vi "processamento_deteccao_frequencia_natural_vibracao.vi"() -> ()   [LabVIEW 2011]
uses:
  <vilib>/measure/NI_MAPro.lvlib
  <vilib>/measure/mamon.llb/Waveform Peak Detection for 1 Chan.vi
  <vilib>/measure/maspectr.llb/FFT Spectrum (Mag-Phase) for 1 Chan.vi
panel:
  out "x/y":dbl[](array[numeric])
  in  "Coluna":i32
  out "x-y":dbl
  out "direito 2":dbl
  out "esquerdo 2":dbl
  in  "Frequência de amostragem":dbl
  out "?":waveform(dbl)(graph)
  out "direito":dbl
  out "esquerdo":dbl
  out "Espectro de frequência (detalhado)":cluster{"Y":dbl[], "Y":dbl[]}[](graph)
  out "Picos de frequência\n(frequência, amplitude)":dbl[][](array[numeric])
  out "Espectro de frequência":cluster{"f0":dbl, "df":dbl, "magnitude":dbl[]}(graph)
  in  "stop":bool
  in  "Abrir arquivo":path
  # "PROGRAMA DE IDENTIFICAÇÃO DE \nFREQUÊNCIA NATURAL DE VIBRAÇÃO"
  # "Desenvolvido por\nEloi Antonio Triaca"
  # "*É recomendável que o cursor esquerdo (amarelo) permaneça na posição \"X =0\" ."
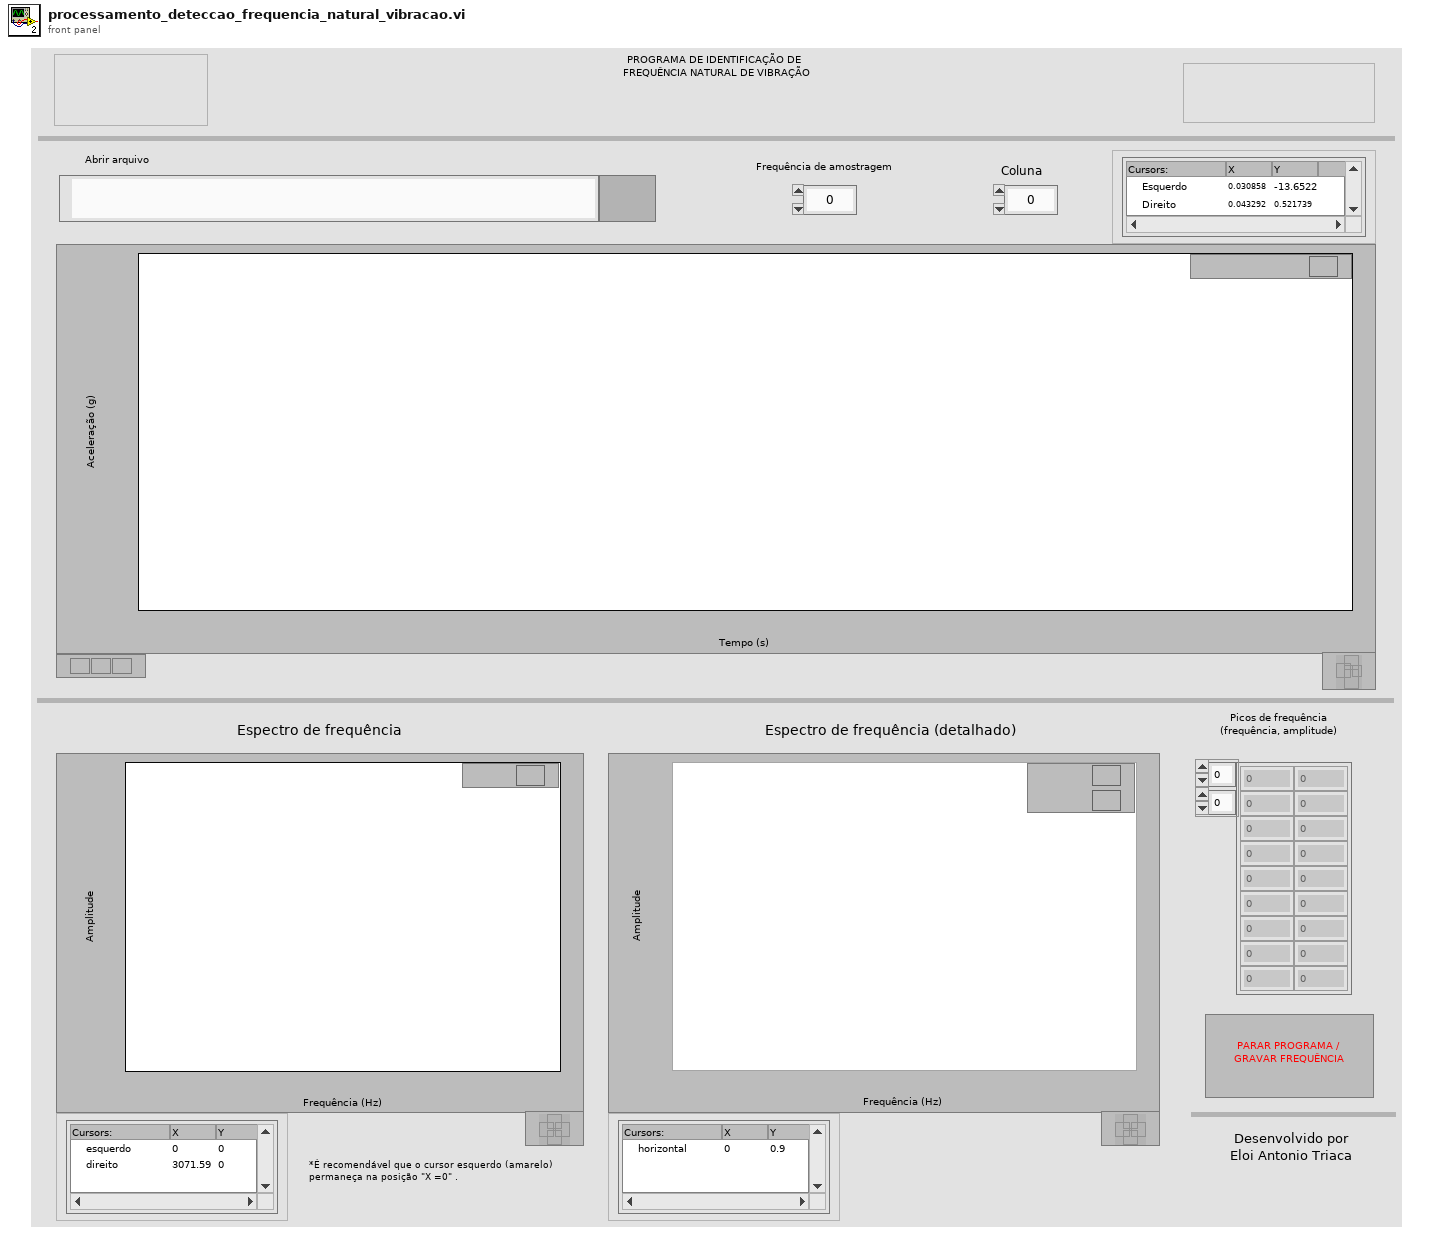
[diagram p1: front panel]
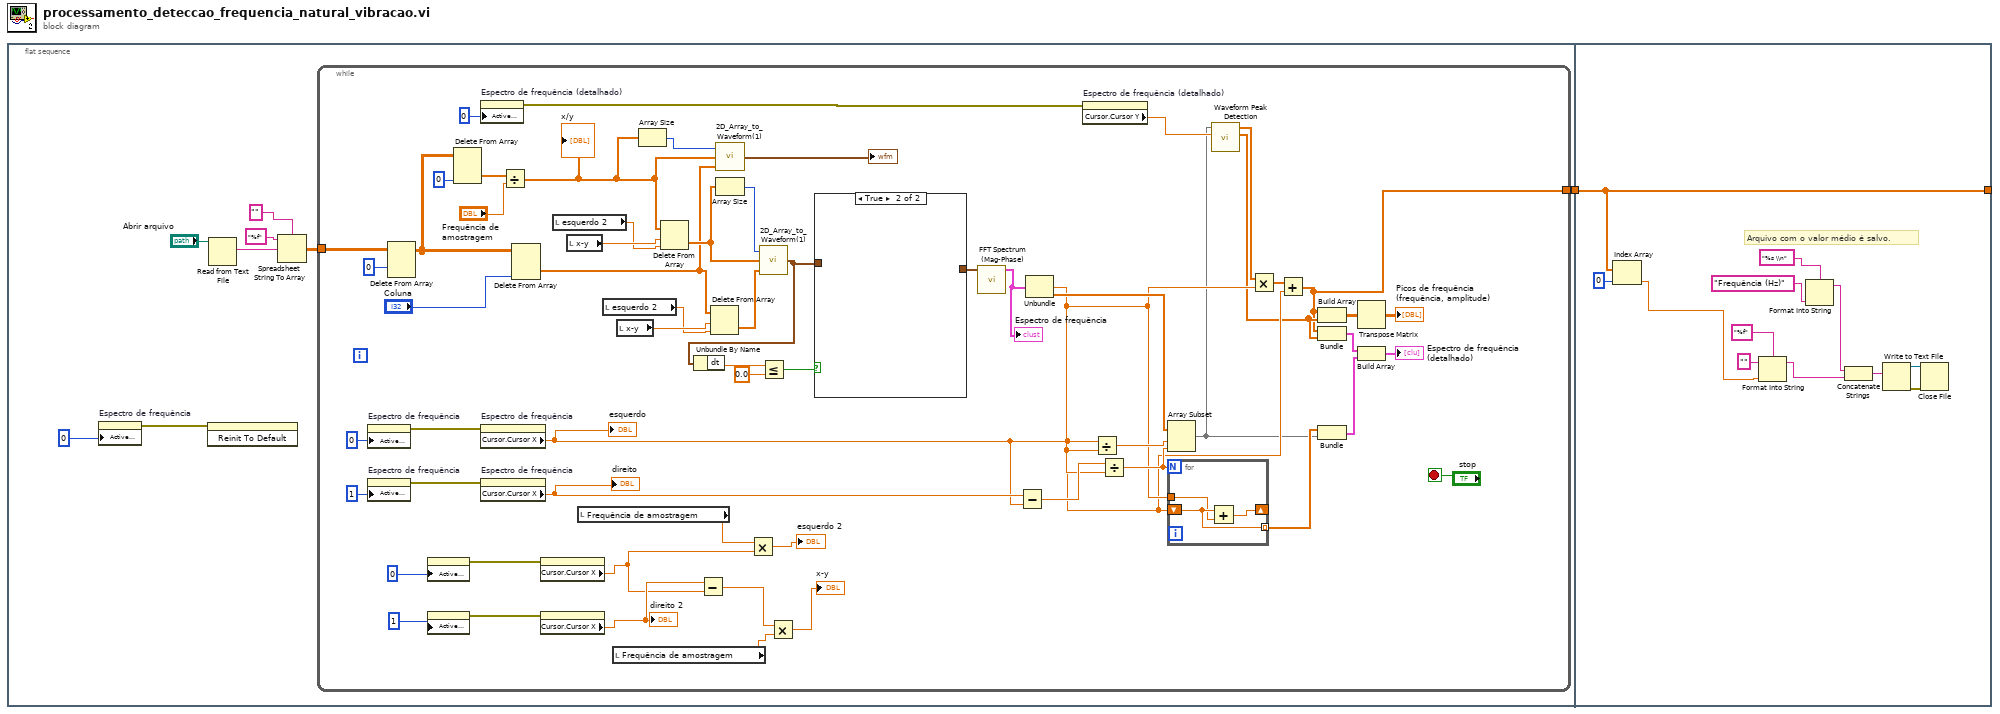
[diagram p0: block diagram]
diagram:
  n1 = flat-sequence {
    tunnel: [w9] -> w1
    tunnel: [w77] -> _
    tunnel: w1 -> [w77]
    frame #0 {
      n2 = property on="Espectro de frequência" class="WFGraph (strict)"("Active Cursor"=u32 0) -> (error out=w2:errorcluster)  [unwired: 2 in, 1 out]
      n3 = invoke class="WFGraph (strict)" method="Reinit To Default"(error in=w2) -> ()  [unwired: 2 in, 3 out]
      n4 = Read from Text File(file (use dialog)="Abrir arquivo") -> (text=w5:string)  [unwired: 3 in, 3 out]
      n5 = Spreadsheet String To Array(delimiter (Tab)="", format string="%f", spreadsheet string=w5) -> (array=w4:dbl[][])  [unwired: 1 in]
      n6 = while {
        tunnel: w4 -> [w69]
        tunnel: [w18] -> w9
        stop <- "stop" stop-if-true
        n7 = property on="Espectro de frequência" class="WFGraph (strict)"("Active Cursor"=u32 0) -> (error out=w62:errorcluster)  [unwired: 2 in, 1 out]
        n8 = property on="Espectro de frequência" class="WFGraph (strict)"("Active Cursor"=u32 1) -> (error out=w61:errorcluster)  [unwired: 2 in, 1 out]
        n9 = Delete From Array(array=w69, index (row)=0) -> (array with subset deleted=w66:dbl[][])  [unwired: 2 in, 1 out]
        n10 = property class="WFGraph (strict)"("Active Cursor"=u32 0) -> (error out=w40:errorcluster)  [unwired: 2 in, 1 out]
        n11 = property class="WFGraph (strict)"("Active Cursor"=u32 1) -> (error out=w39:errorcluster)  [unwired: 2 in, 1 out]
        n12 = Delete From Array(array=w66, index (col)=0) -> (deleted portion=w44:dbl[])  [unwired: 2 in, 1 out]
        n13 = property on="Espectro de frequência (detalhado)" class="XYGraph (strict)"("Active Cursor"=u32 0) -> (error out=w47:errorcluster)  [unwired: 2 in, 1 out]
        n14 = property on="Espectro de frequência" class="WFGraph (strict)"(error in=w62) -> ("Cursor.Cursor X"=w45:dbl)  [unwired: 1 in, 2 out]
        "esquerdo" <- w45
        n15 = property on="Espectro de frequência" class="WFGraph (strict)"(error in=w61) -> ("Cursor.Cursor X"=w60:dbl)  [unwired: 1 in, 2 out]
        "direito" <- w60
        n16 = Divide(x=w44, y="Frequência de amostragem") -> (x/y=w23:dbl[])
        "x/y" <- w23
        n17 = Delete From Array(array=w66, index (col)="Coluna") -> (deleted portion=w24:dbl[])  [unwired: 2 in, 1 out]
        n18 = property class="WFGraph (strict)"(error in=w40) -> ("Cursor.Cursor X"=w25:dbl)  [unwired: 1 in, 2 out]
        n19 = property class="WFGraph (strict)"(error in=w39) -> ("Cursor.Cursor X"=w38:dbl)  [unwired: 1 in, 2 out]
        "direito 2" <- w38
        n20 = local read "esquerdo 2"() -> (w33:dbl)
        n21 = local read "x-y"() -> (w34:dbl)
        n22 = local read "Frequência de amostragem"() -> (w26:dbl)
        n23 = local read "esquerdo 2"() -> (w31:dbl)
        n24 = local read "Frequência de amostragem"() -> (w30:dbl)
        n25 = local read "x-y"() -> (w32:dbl)
        n26 = Array Size(array=w23) -> (size(s)=w22:i32)
        n27 = Delete From Array(array=w23, length=w34, index=w33) -> (deleted portion=w36:dbl[])  [unwired: 1 out]
        n28 = Subtract(x=w38, y=w25) -> (x-y=w29:dbl)
        n29 = Delete From Array(array=w24, length=w32, index=w31) -> (deleted portion=w35:dbl[])  [unwired: 1 out]
        n30 = call "2D_Array_to_Waveform(1).vi"("Y"=w24, "X"=w23, "Nº de amostras"=w22) -> ("output waveform"=→"?":waveform(dbl))
        n31 = Array Size(array=w36) -> (size(s)=w37:i32)
        n32 = Multiply(x=w26, y=w25) -> (x*y=→"esquerdo 2":dbl)
        n33 = call "2D_Array_to_Waveform(1).vi"("Y"=w35, "X"=w36, "Nº de amostras"=w37) -> ("output waveform"=w13:waveform(dbl))
        n34 = Unbundle By Name(w13) -> ("dt"=w15:dbl)
        n35 = Less Or Equal?(x=w15, y=0.0) -> (x <= y?=w11:bool)
        n36 = Multiply(x=w29, y=w30) -> (x*y=→"x-y":dbl)
        n37 = case shown="True" w11 {
          tunnel: w13 -> [w71 _]
          tunnel: [w71 _] -> w12
          frame False {
          }
          frame True {
          }
        }
        n38 = call-poly <vilib>:"FFT Spectrum (Mag-Phase).vi"("time signal"=w12) -> ("magnitude"=w16:cluster{"f0":dbl, "df":dbl, "magnitude":dbl[]})  [unwired: 6 in, 4 out]
        "Espectro de frequência" <- w16
        n39 = Subtract(x=w60, y=w45) -> (x-y=w59:dbl)
        n40 = Unbundle(w16) -> ("df"=w55:dbl, "magnitude"=w65:dbl[])  [unwired: 1 out]
        n41 = property on="Espectro de frequência (detalhado)" class="XYGraph (strict)"(error in=w47) -> ("Cursor.Cursor Y"=w46:dbl)  [unwired: 1 in, 2 out]
        n42 = Divide(x=w45, y=w55) -> (x/y=w58:dbl)
        n43 = Divide(x=w59, y=w55) -> (x/y=w56:dbl)
        n44 = Array Subset(array=w65, index=w58, length=w56) -> (w10:dbl[])
        n45 = for {
          N: w56 -> [_]
          shift-right: [w74] -> _
          shift-left: w45 -> [w73]
          tunnel: [w73] -> w54 mode=indexing
          tunnel: w55 -> [w72]
          n46 = Add(x=w73, y=w72) -> (x+y=w74:dbl)
        }
        n47 = call-poly <vilib>:"Waveform Peak Detection.vi"("threshold"=w46, "Signal In"=w10) -> ("Amplitudes"=w19:dbl[], "Locations"=w20:dbl[])  [unwired: 5 in, 3 out]
        n48 = Multiply(x=w20, y=w55) -> (x*y=w57:dbl[])
        n49 = Add(x=w57, y=w45) -> (x+y=w18:dbl[])
        n50 = Build Array(w18, w19) -> (w53:dbl[][])
        n51 = Bundle(w18, "Amplitudes"=w19) -> (w51:cluster{dbl[], "Amplitudes":dbl[]})  [unwired: 1 in]
        n52 = Bundle(w54, w10) -> (w50:cluster{dbl[], dbl[]})  [unwired: 1 in]
        n53 = Transpose Matrix(1:w53) -> (0:→"Picos de frequência\n(frequência, amplitude)":dbl[][])
        n54 = Build Array(w51, w50) -> (→"Espectro de frequência (detalhado)":cluster{dbl[], "Amplitudes":dbl[]}[])
      }
    }
    frame #1 {
      # "Arquivo com o valor médio é salvo."
      n55 = Index Array(array=w77, index=0) -> (element=w75:dbl)
      n56 = Format Into String(format string="%f", initial string="", w75) -> (resulting string=w79:string)  [unwired: 1 in, 1 out]
      n57 = Format Into String(format string="%s \\n", "Frequência (Hz)" ("input 1")) -> (resulting string=w84:string)  [unwired: 2 in, 1 out]
      n58 = Concatenate Strings(w84, w79) -> (w81:string)
      n59 = Write to Text File(text=w81) -> (refnum out=w83:refnum<file>, error out=w82:errorcluster)  [unwired: 3 in, 1 out]
      n60 = Close File(refnum=w83, error in=w82) -> ()  [unwired: 2 out]
    }
  }
